vi "camera.vi"() -> ()   [LabVIEW 2020]
uses:
  <vilib>/userDefined/High Color/IMAQdx.ctl
  <vilib>/vision/driver/NI_Vision_Acquisition_Software.lvlib
panel:
  in  "Tab Control":enum32{"Snap", "Grab"}(tab)
  in  "Camera Select 1":T1
  out "Image":T2(plugin-control)
  out "error out":errorcluster
  in  "Camera Select 2":T1
  out "Image 2":T2(plugin-control)
  out "Buffer Number Out":u32
  in  "종료버튼":bool
  out "x/y":dbl
  in  "동영상을 저장":bool
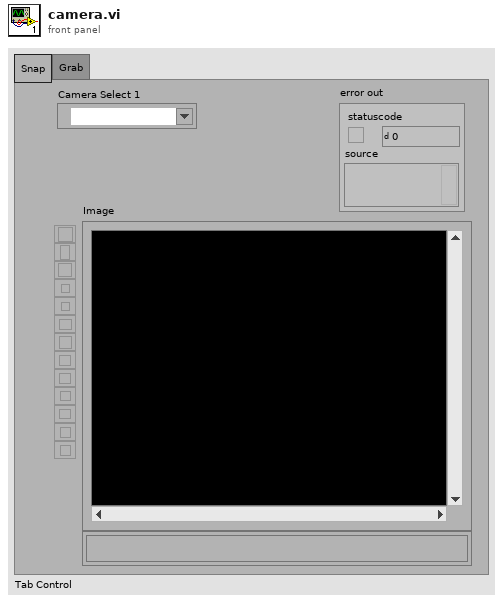
[diagram p1: front panel]
types:
  T1 = typedef "IMAQdx.ctl" = refnum<k21>
  T2 = typedef "IMAQ Image.ctl" = refnum<image>
  T3 = typedef "IMAQ AVI2 Refnum.ctl" = refnum<k20>
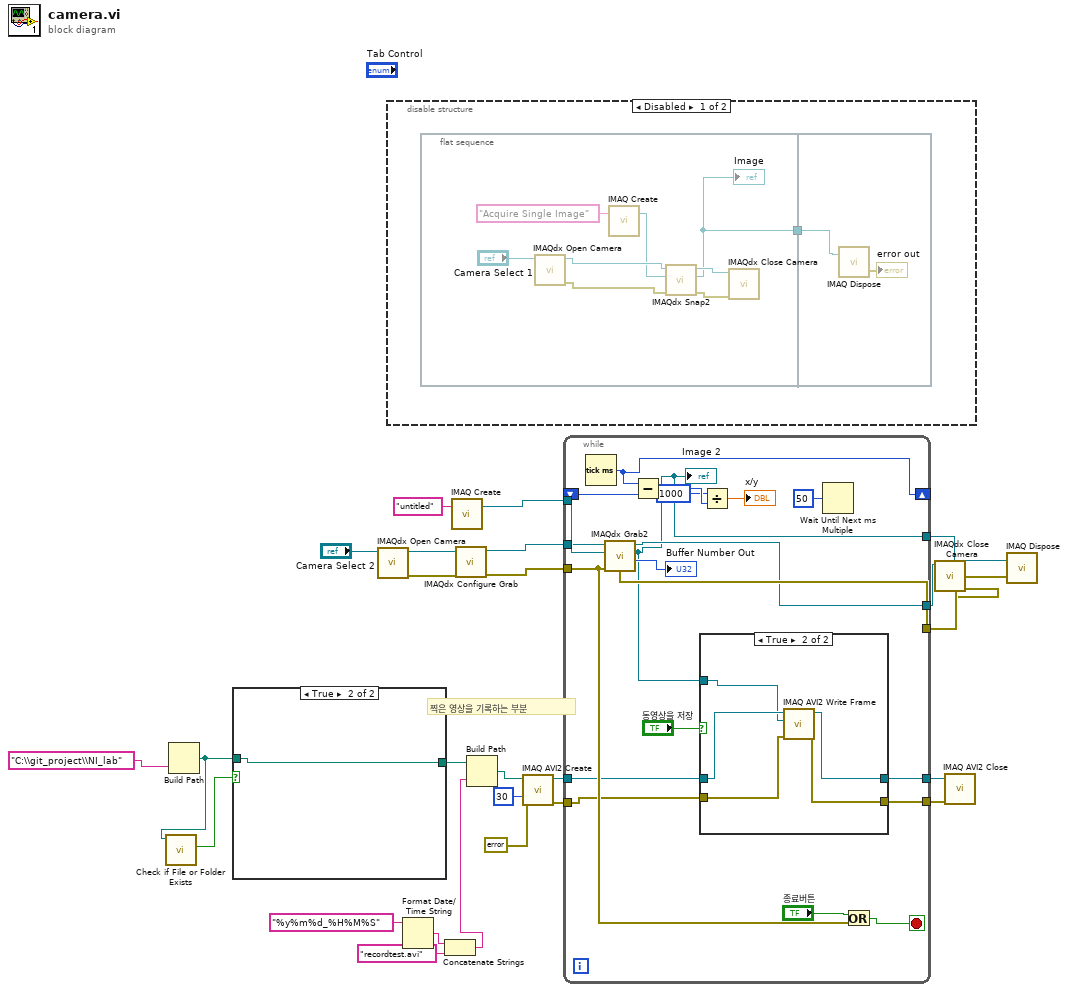
[diagram p0: block diagram]
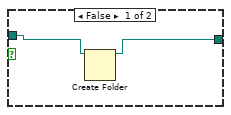
[diagram p2: hidden frame]
diagram:
  # "찍은 영상을 기록하는 부분"
  n1 = Build Path(name or relative path="C:\\git_project\\NI_lab") -> (appended path=w14:path)  [unwired: 1 in]
  n2 = call <vilib>:"Check if File or Folder Exists.vi"("path"=w14) -> ("file or folder exists?"=w13:bool)  [unwired: 8 in, 2 out]
  n3 = case shown="True" w13 {
    tunnel: w14 -> [w28 w29]
    tunnel: [w27 w29] -> w1
    frame False {
      n4 = Create Folder(path (use dialog)=w28) -> (created path=w27:path)  [unwired: 2 in, 2 out]
    }
    frame True {
    }
  }
  n5 = call <vilib>:"IMAQdx Open Camera.vi"("Session In"="Camera Select 2") -> ("error out"=w23:errorcluster, "Session Out"=w24:T1)  [unwired: 9 in]
  n6 = disable-structure shown="Disabled" {
    frame Disabled {
      n7 = flat-sequence {
        tunnel: [w32] -> w30
        tunnel: w30 -> [w39]
        frame #0 {
          n8 = call <vilib>:"IMAQdx Open Camera.vi"("Session In"="Camera Select 1") -> ("error out"=w35:errorcluster, "Session Out"=w36:T1)  [unwired: 9 in]
          n9 = call "IMAQ Create"("Image Name"="Acquire Single Image") -> ("New Image"=w33:T2)  [unwired: 4 in, 1 out]
          n10 = call <vilib>:"IMAQdx Snap2.vi"("error in"=w35, "Image In"=w33, "Session In"=w36) -> ("error out"=w31:errorcluster, "Image Out"=w32:T2, "Session Out"=w34:T1)  [unwired: 6 in]
          "Image" <- w32
          n11 = call <vilib>:"IMAQdx Close Camera.vi"("error in"=w31, "Session In"=w34) -> ()  [unwired: 9 in, 1 out]
        }
        frame #1 {
          n12 = call "IMAQ Dispose"("Image"=w39) -> ("error out"=→"error out":errorcluster)  [unwired: 5 in]
        }
      }
    }
    frame Enabled {
    }
  }
  n13 = Format Date/Time String(time format string (%c)="%y%m%d_%H%M%S") -> (date/time string=w17:string)  [unwired: 2 in]
  n14 = Concatenate Strings(w17, "recordtest.avi" ("string")) -> (w16:string)
  n15 = call "IMAQ Create"("Image Name"="untitled") -> ("New Image"=w22:T2)  [unwired: 4 in, 1 out]
  n16 = call <vilib>:"IMAQdx Configure Grab.vi"("error in"=w23, "Session In"=w24) -> ("error out"=w20:errorcluster, "Session Out"=w21:T1)  [unwired: 8 in]
  n17 = Build Path(base path=w1, name or relative path=w16) -> (appended path=w11:path)
  n18 = call "IMAQ AVI2 Create"("error in (no error)"=errorcluster {"status"=FALSE, "code"=0, "source"=""}, "Frames Per Second"=u32 30, "AVI Path"=w11) -> ("error out"=w8:errorcluster, "AVI Refnum"=w7:T3)  [unwired: 7 in]
  n19 = while {
    tunnel: w22 -> [w60]
    tunnel: w21 -> [w59]
    tunnel: w20 -> [w58]
    tunnel: [w41] -> w19
    shift-right: [w53] -> _
    shift-left: _ -> [w54]
    tunnel: w8 -> [w46]
    tunnel: w7 -> [w47]
    tunnel: [w45] -> w6
    tunnel: [w44] -> w5
    tunnel: [w43] -> w4
    tunnel: [w42] -> w3
    stop <- w56 stop-if-true
    n20 = Tick Count (ms)() -> (millisecond timer value=w53:u32)
    n21 = call <vilib>:"IMAQdx Grab2.vi"("error in"=w58, "Image In"=w60, "Session In"=w59) -> ("error out"=w43:errorcluster, "Buffer Number Out"=→"Buffer Number Out":u32, "Image Out"=w41:T2, "Session Out"=w42:T1)  [unwired: 5 in]
    "Image 2" <- w41
    n22 = Subtract(x=w53, y=w54) -> (x-y=w52:u32)
    n23 = case shown="True" "동영상을 저장" {
      tunnel: w41 -> [_ w63]
      tunnel: w47 -> [w62 w67]
      tunnel: w46 -> [w61 w65]
      tunnel: [w62 w66] -> w45
      tunnel: [w61 w64] -> w44
      frame False {
      }
      frame True {
        n24 = call "IMAQ AVI2 Write Frame"("error in (no error)"=w65, "Image"=w63, "AVI Refnum"=w67) -> ("error out"=w64:errorcluster, "AVI Refnum (duplicate)"=w66:T3)  [unwired: 6 in, 1 out]
      }
    }
    n25 = Divide(x=u32 1000, y=w52) -> (x/y=→"x/y":dbl)
    n26 = Wait Until Next ms Multiple(millisecond multiple=u32 50) -> ()  [unwired: 1 out]
    n27 = Or(x="종료버튼", y=w58) -> (x .or. y?=w56:bool)
  }
  n28 = call <vilib>:"IMAQdx Close Camera.vi"("error in"=w4, "Session In"=w3) -> ("error out"=w2:errorcluster)  [unwired: 9 in]
  n29 = call "IMAQ AVI2 Close"("error in (no error)"=w5, "AVI Refnum"=w6) -> ()  [unwired: 9 in, 1 out]
  n30 = call "IMAQ Dispose"("Image"=w19, "error in (no error)"=w2) -> ()  [unwired: 4 in, 1 out]
